vi "RT_wait.vi"(3 "Counter Units":u16(ring)=2 items=["Ticks", "uSec", "mSec"], 4 "Count(mSec)":u32, 5 "error in (no error)":errorcluster) -> (0 "Tick Count(mSec)":u32, 1 "error out":errorcluster)   [LabVIEW 2016]
doc: "Waits until the value of the timer becomes a multiple of <B>Count</B>. Use this function to synchronize activities. You can call this function in a loop to control the loop execution rate."
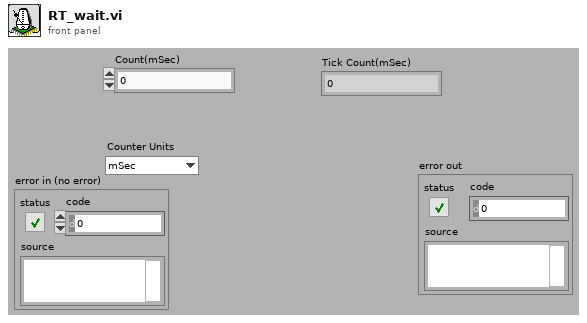
[diagram p1: front panel]
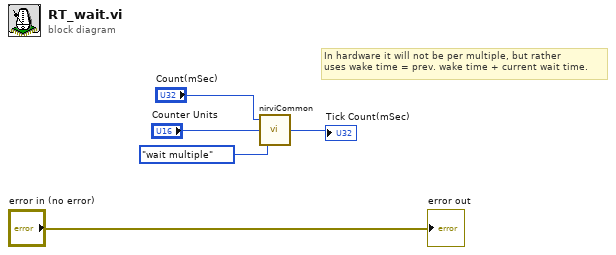
[diagram p0: block diagram]
diagram:
  # "In hardware it will not be per multiple, but rather\nuses wake time = prev. wake time + current wait time."
  n1 = call <vilib>:"nirviCommon.vi"("Action"=enum16{"wait", "wait multiple", "tick count"}."wait multiple", "Counter Units"="Counter Units", "Count(uSec)"="Count(mSec)") -> ("Tick Count(uSec)"=→"Tick Count(mSec)":u32)
  "error out" <- "error in (no error)"
